vi "Initialize.vi"(5 "error in (no error)":errorcluster) -> (14 "image out":refnum<class "MSC Image.lvclass">, 19 "error out":errorcluster)   [LabVIEW 2014, in "MSC Image.lvclass"]
doc: "Initializes an image and loads \"NA.png\" as a placeholder."
uses:
  MSC Image.lvclass
  controls/Image.ctl
  controls/Size.ctl
  controls/Image Type.ctl
  MSC Image.lvclass/MSC Image.ctl
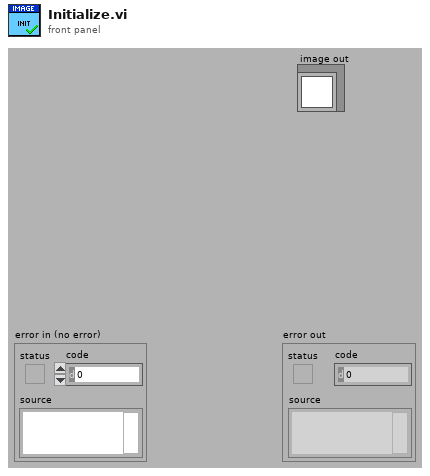
[diagram p1: front panel]
types:
  T1 = typedef "MSC Image.lvclass/Image.ctl" = cluster{"Pointer":u64, "Size":T2, "Image Type":T3, "Time Stamp":timestamp, "Variant":variant}
  T2 = typedef "MSC Image.lvclass/Size.ctl" = cluster{"Cols":i32, "Rows":i32}
  T3 = typedef "MSC Image.lvclass/Image Type.ctl" = i32
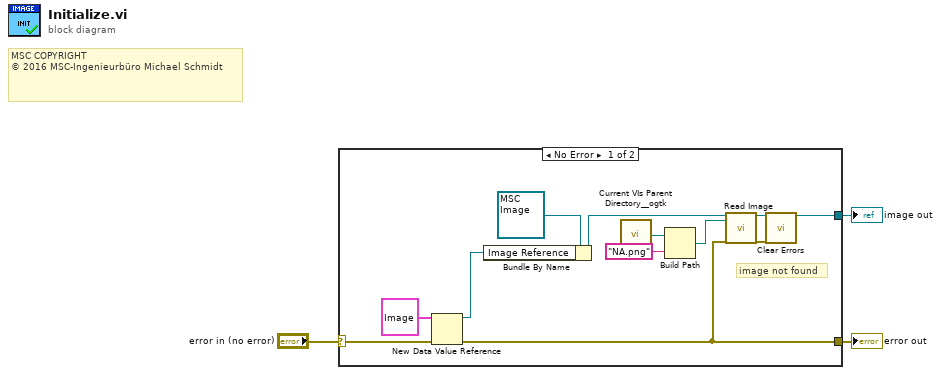
[diagram p0: block diagram]
diagram:
  # "MSC COPYRIGHT\n© 2016 MSC-Ingenieurbüro Michael Schmidt"
  n1 = case shown="No Error" "error in (no error)" {
    selector: "error in (no error)" -> [w13 w15]
    tunnel: [w7 _] -> w3
    tunnel: [w5 w15] -> w1
    frame No Error {
      # "image not found"
      n2 = New Data Value Reference(data value=T1 {"Pointer"=0, "Size"={"Cols"=0, "Rows"=0}, "Image Type"=0, "Time Stamp"=timestamp(0 s since 1904-01-01), "Variant"=variant} ("Image"), error in=w13) -> (data value reference=w12:refnum<data-value>, error out=w5:errorcluster)
      n3 = Bundle By Name(cluster=refnum<class "MSC Image.lvclass"> refnum ("image out"), "Image Reference"=w12) -> (w9:refnum<class "MSC Image.lvclass">)
      n4 = call <userlib>:"Current VIs Parent Directory__ogtk.vi"() -> ("Parent Directory (+ Relative)"=w11:path)  [unwired: 5 in]
      n5 = Build Path(base path=w11, name or relative path="NA.png") -> (appended path=w8:path)
      n6 = call-dynamic "Read Image.vi"("image in"=w9, "image path"=w8, "error in (no error)"=w5) -> ("image out"=w7:refnum<class "MSC Image.lvclass">, "error out"=w6:errorcluster)  [unwired: 15 in]
      n7 = call <vilib>:"Clear Errors.vi"("error in (no error)"=w6) -> ()  [unwired: 5 in, 2 out]
    }
    frame Error {
    }
  }
  "image out" <- w3
  "error out" <- w1
